vi "FileDelete.vi"(8 "error in (no error)":errorcluster, 9 "Silent?":bool, 10 "(Empty=No Action)":path caption="File to Delete", 11 "controller in":refnum<k24>) -> (0 "error out":errorcluster, 3 "controller out":refnum<k24>)   [LabVIEW 2010]
uses:
  c:/aerotech/controller/5.xx.xxx/ensemble/pc/labview/2010/bin/Aerotech.Ensemble.dll
  bin/Aerotech.Ensemble.dll
  c:/aerotech/controller/5.xx.xxx/ensemble/pc/labview/2010/bin/Aerotech.Ensemble.LabVIEW.dll
  bin/Aerotech.Ensemble.LabVIEW.dll
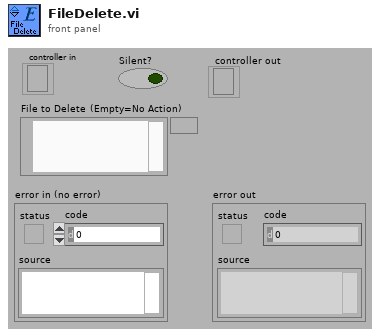
[diagram p1: front panel]
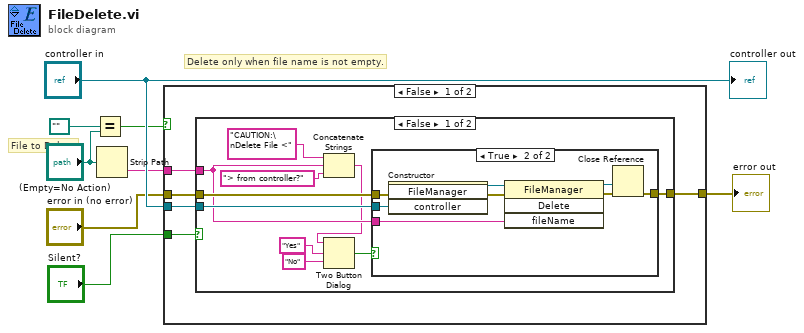
[diagram p0: block diagram]
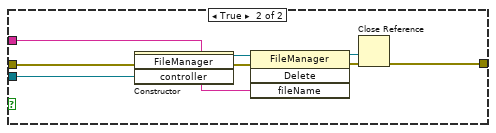
[diagram p3: hidden frame]
diagram:
  # "File to Delete"
  # "Delete only when file name is not empty."
  n1 = Equal?(x=path "", y="(Empty=No Action)") -> (x = y?=w5:bool)
  n2 = Strip Path(path="(Empty=No Action)") -> (name=w2:string)  [unwired: 1 out]
  n3 = case shown="False" w5 {
    tunnel: [w13 w41] -> w8
    tunnel: "error in (no error)" -> [w12 w41]
    tunnel: "controller in" -> [w11 _]
    tunnel: w2 -> [w10 _]
    tunnel: "Silent?" -> [w9 _]
    frame False {
      n4 = case shown="False" w9 {
        tunnel: [w23 w38] -> w13
        tunnel: w12 -> [w22 w36]
        tunnel: w11 -> [w21 w35]
        tunnel: w10 -> [w19 w33]
        frame False {
          n5 = Concatenate Strings("CAUTION:\nDelete File <" ("message"), w19, "> from controller?" ("string")) -> (w17:string)
          n6 = Two Button Dialog(message=w17, 1:"No" ("F button name (\"Cancel\")"), 2:"Yes" ("T button name (\"OK\")")) -> (T button?=w14:bool)
          n7 = case shown="True" w14 {
            tunnel: [w24 w30] -> w23
            tunnel: w22 -> [w24 w28]
            tunnel: w21 -> [_ w27]
            tunnel: w19 -> [_ w25]
            frame False {
            }
            frame True {
              n8 = constructor class="FileManager"(error in=w28, "controller"=w27) -> (reference out=w26:refnum<k24>, error out=w29:errorcluster)  [unwired: 2 in, 2 out]
              n9 = invoke class="FileManager" method="Delete"(reference=w26, error in=w29, "fileName"=w25) -> (reference out=w31:refnum<k24>, error out=w32:errorcluster)  [unwired: 1 in, 2 out]
              n10 = Close Reference(reference=w31, error in (no error)=w32) -> (error out=w30:errorcluster)
            }
          }
        }
        frame True {
          n11 = constructor class="FileManager"(error in=w36, "controller"=w35) -> (reference out=w34:refnum<k24>, error out=w37:errorcluster)  [unwired: 2 in, 2 out]
          n12 = invoke class="FileManager" method="Delete"(reference=w34, error in=w37, "fileName"=w33) -> (reference out=w39:refnum<k24>, error out=w40:errorcluster)  [unwired: 1 in, 2 out]
          n13 = Close Reference(reference=w39, error in (no error)=w40) -> (error out=w38:errorcluster)
        }
      }
    }
    frame True {
    }
  }
  "error out" <- w8
  "controller out" <- "controller in"
